vi "NewStep.vi"(9 "Step":dbl, 10 "Max":dbl format="%#_13g", 11 "Current Value":dbl format="%#_13g") -> (3 "Step 2":dbl)   [LabVIEW 2018]
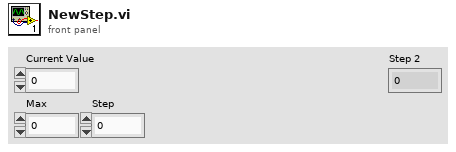
[diagram p1: front panel]
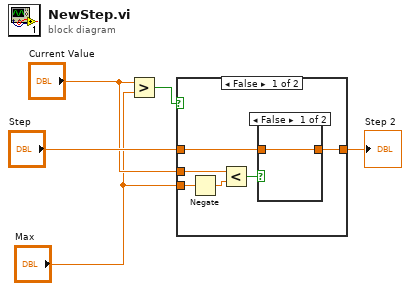
[diagram p0: block diagram]
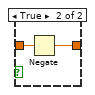
[diagram p2: hidden frame]
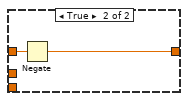
[diagram p3: hidden frame]
diagram:
  n1 = Greater?(x="Current Value", y="Max") -> (0:w5:bool)
  n2 = case shown="False" w5 {
    tunnel: "Step" -> [w8 w16]
    tunnel: "Current Value" -> [w11 _]
    tunnel: "Max" -> [w10 _]
    tunnel: [w7 w15] -> w1
    frame False {
      n3 = Negate(x=w10) -> (-x=w9:dbl)
      n4 = Less?(x=w11, y=w9) -> (x < y?=w6:bool)
      n5 = case shown="False" w6 {
        tunnel: w8 -> [w12 w14]
        tunnel: [w12 w13] -> w7
        frame False {
        }
        frame True {
          n6 = Negate(x=w14) -> (-x=w13:dbl)
        }
      }
    }
    frame True {
      n7 = Negate(x=w16) -> (-x=w15:dbl)
    }
  }
  "Step 2" <- w1
